vi "Data Access.vi"(8 "error in (no error)":errorcluster, 10 "Data Access Handler":refnum<class "Data Access Handler.lvclass">, 11 "Flex Msg in":refnum<class "Open File Msg.lvclass">) -> (0 "error out":errorcluster, 3 "Flex Msg out":refnum<class "Open File Msg.lvclass">)   [LabVIEW 2020, in "File Writer.lvlib" / "Open File Msg.lvclass"]
doc: "Expose class private data to the front panel while letting the Data Access Handler class act on the data."
uses:
  Open File Msg.lvclass
  C:/Current projects/WS/PPL/HDH.Actor Framework.Core.Msg.lvlibp/Flex Msg/Flex Msg.lvclass
  PPL/HDH.Actor Framework.Core.Msg.lvlibp/Flex Msg/Data Access Handlers/Data Access Handler/Data Access Handler.lvclass
  Open File Msg.lvclass/Open File Msg.ctl
panel:
  in  "Await Completion?":bool
  in  "New Path":path
  in  "Cancel":bool
  in  "OK":bool
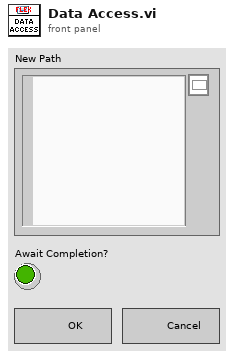
[diagram p1: front panel]
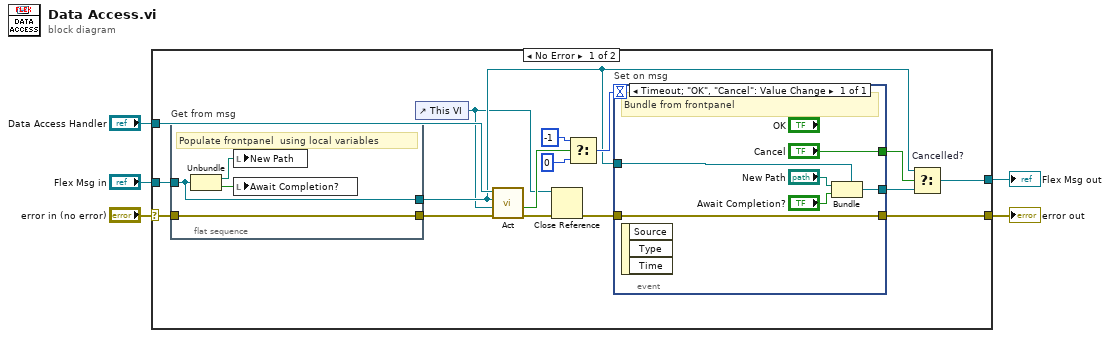
[diagram p0: block diagram]
diagram:
  n1 = case shown="No Error" "error in (no error)" {
    selector: "error in (no error)" -> [w21 w33]
    tunnel: [w14 w33] -> w4
    tunnel: [w9 w32] -> w2
    tunnel: "Flex Msg in" -> [w12 w32]
    tunnel: "Data Access Handler" -> [w20 _]
    frame No Error {
      n2 = flat-sequence "Get from msg" {
        tunnel: w21 -> [w31]
        tunnel: [w30] -> w7
        tunnel: w12 -> [w30]
        tunnel: [w31] -> w19
        frame #0 {
          # "Populate frontpanel  using local variables"
          n3 = Unbundle(w30) -> (w29:path, w28:bool)
          n4 = local write "New Path"(w29) -> ()
          n5 = local write "Await Completion?"(w28) -> ()
        }
      }
      n6 = control-ref of="This VI"() -> (w6:refnum<vi>)
      n7 = call-dynamic "Act.vi"("error in (no error)"=w19, "VI Refnum in"=w6, "Flex Msg type"=w7, "Data Access Handler in"=w20) -> ("error out"=w11:errorcluster, "Await user action?"=w18:bool)  [unwired: 5 in, 1 out]
      n8 = Close Reference(reference=w6, error in (no error)=w11) -> (error out=w13:errorcluster)
      n9 = Select(t=-1, s=w18, f=0 ("t")) -> (s? t:f=w15:i32)
      n10 = event "Set on msg" shown="[0] Timeout;  \"OK\", \"Cancel\": Value Change" {
        selector: _ -> [_]
        dyn-events: _ -> [_]
        timeout: w15 -> [_]
        tunnel: [w27] -> w14
        tunnel: w13 -> [w27]
        tunnel: ["Cancel"] -> w10
        tunnel: [w24] -> w8
        tunnel: w7 -> [w26]
        event Timeout; "OK", "Cancel": Value Change {
          # "Bundle from frontpanel"
          n11 = event-data() -> ()  [unwired: 1 in, 3 out]
          n12 = Bundle(cluster=w26, "New Path", "Await Completion?") -> (w24:refnum<class "Open File Msg.lvclass">)
        }
      }
      n13 = Select "Cancelled?"(t=w7, s=w10, f=w8) -> (s? t:f=w9:refnum<class "Open File Msg.lvclass">)
    }
    frame Error {
    }
  }
  "error out" <- w4
  "Flex Msg out" <- w2
